vi "Read Headers.vi"(8 "Error In":errorcluster, 11 "DVR In":refnum<data-value>) -> (0 "Error Out":errorcluster, 2 "Start End Dates":T1, 3 "DVR Out":refnum<data-value>, 5 "AE Owner String":string[](array[string]), 7 "SR Status String":string[](array[string]))   [LabVIEW 2016, in "Data Operations.lvlib"]
uses:
  Data Operations.lvlib
  Private Controls/Report Data Cluster.ctl
  Private Controls/Data Raw.ctl
  Public Controls/Start End Date Cluster.ctl
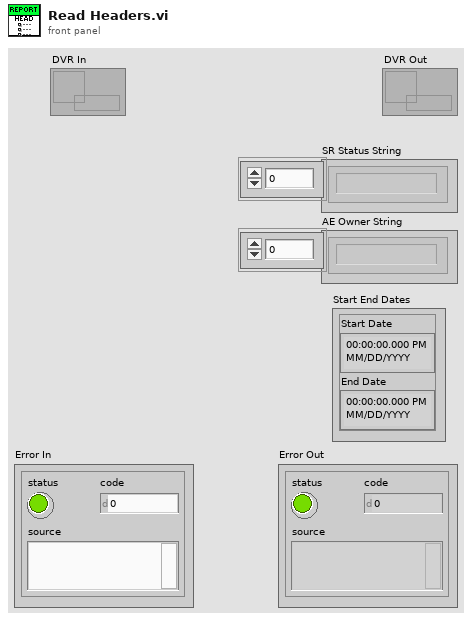
[diagram p1: front panel]
types:
  T1 = typedef "Data Operations.lvlib/Start End Date Cluster.ctl" = cluster{"Start Date":timestamp, "End Date":timestamp}
  T2 = typedef "Data Operations.lvlib/Report Data Cluster.ctl" = cluster{"Headers":cluster{"Start Date":timestamp, "End Date":timestamp, "SR Status String":string[], "AE Owner String":string[]}, "Data":T3[]}
  T3 = typedef "Data Operations.lvlib/Data Raw.ctl" = cluster{"SR Number":string, "Status":string, "Summary":string, "AE Owner":string, "AE Group":string, "SurveyData":cluster{"Resolution Time":dbl, "Total Satisfaction":dbl, "Response Time":dbl, "Courtesy":dbl, "Problem Solved":dbl}, "Time Data":cluster{"Last Update Date":timestamp, "Request Date":timestamp, "Request week":u8}}
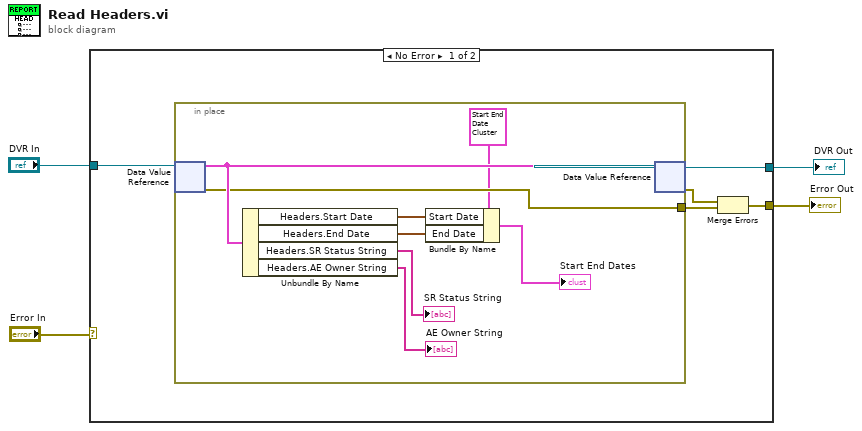
[diagram p0: block diagram]
diagram:
  n1 = case shown="No Error" "Error In" {
    selector: "Error In" -> [_ w19]
    tunnel: "DVR In" -> [w9 w18]
    tunnel: [w7 w19] -> w3
    tunnel: [w6 w18] -> w1
    frame No Error {
      n2 = in-place {
        in-place-border: [w14] -> w8
        n3 = in-place-dvr #1(w9) -> (w17:T2, w14:errorcluster)
        n4 = Unbundle By Name(w17) -> ("Headers.Start Date"=w12:timestamp, "Headers.End Date"=w11:timestamp, "Headers.SR Status String"=→"SR Status String":string[], "Headers.AE Owner String"=→"AE Owner String":string[])
        n5 = Bundle By Name(cluster=T1 {"Start Date"=timestamp(3566070001 s since 1904-01-01), "End Date"=timestamp(3568834799 s since 1904-01-01)} ("Cluster"), "Start Date"=w12, "End Date"=w11) -> (→"Start End Dates":T1)
        n6 = in-place-dvr #1(w17) -> (w6:refnum<data-value>, w5:errorcluster)
      }
      n7 = Merge Errors(w5, w8) -> (w7:errorcluster)
    }
    frame Error {
    }
  }
  "Error Out" <- w3
  "DVR Out" <- w1
